vi "create Timings.vi"(8 "error in (no error)":errorcluster, 10 "Parameters":u32[](array[numeric]), 11 "Störaussendung in":refnum<class "Stoeraussendung.lvclass">) -> (0 "error out":errorcluster, 1 "wait":i32[](array[numeric])=[0, 30000, 0, 0], 2 "timeout":u32[](array[numeric]), 3 "Störaussendung out":refnum<class "Stoeraussendung.lvclass">)   [LabVIEW 2013, in "Stoeraussendung.lvclass"]
uses:
  Stoeraussendung.lvclass
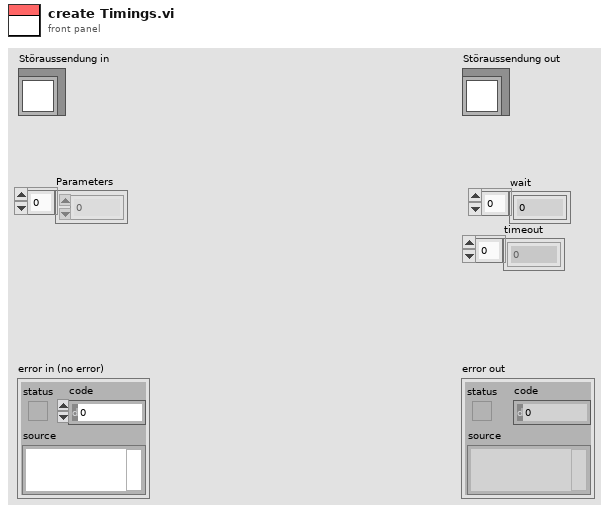
[diagram p1: front panel]
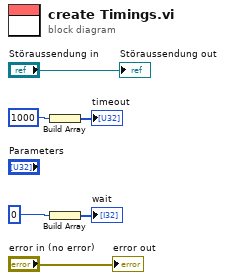
[diagram p0: block diagram]
diagram:
  n1 = Build Array(1000) -> (→"timeout":i32[])
  n2 = Build Array(0) -> (→"wait":i32[])
  "error out" <- "error in (no error)"
  "Störaussendung out" <- "Störaussendung in"
